vi "HEALTH_LABVIEW_V1.vi"() -> (0 "error out":errorcluster)   [LabVIEW 2026]
panel:
  in  "HEATER ON/OFF":bool
  out "ANALOG VOLTAGE 5\nADDRESS 8:\nHEATER TEMPERATURE":dbl(knob) scale=0.0..2.5
  out "Value 5":dbl format="%.6f"
  out "HEATER TEMP (C)":dbl(graph)
  out "ANALOG VOLTAGE 4\nADDRESS 22:\nCOOLANT OUTLET TEMPERATURE":dbl(knob) scale=0.0..2.5
  out "Value 4":dbl format="%.6f"
  out "ANALOG VOLTAGE 3\nADDRESS 20:\nCOOLANT INLET TEMPERATURE":dbl(knob) scale=0.0..2.5
  out "Value 3":dbl format="%.6f"
  out "ANALOG VOLTAGE 2\nADDRESS 18:\nDIFFERENTIAL PRESSURE":dbl(knob) scale=0.0..2.5
  out "Value 2":dbl format="%.6f"
  out "ANALOG VOLTAGE 1\nADDRESS 16:\nABSOLUTE PRESSURE":dbl(knob) scale=0.0..2.5
  out "Error String":string
  out "Value":dbl format="%.6f"
  out "ConnectionType Out":i32
  out "DeviceType Out":i32
  in  "Identifier":string="LJM_idANY"
  in  "ConnectionType":string="LJM_ctANY"
  in  "DeviceType":string="LJM_dtANY"
  # "LJM_dtT4"
  # "LJM_ctUSB"
  # "Common Registers:\nAddress, Name, Type, Read/Write\n0, AIN0, 3, RO\n2, AIN1, 3, RO\n1000, DAC0, 3, RW\n1002, DAC1, 3, RW\n2000, FIO0, 0, RW\n2001, FIO1, 0, RW\n55110, TEST_UINT16, 0, RW\n60000, PRODUCT_ID, 3, RO\n60004, FIRMWARE_VERSION, 3, RO\n60028, SERIAL_NUMBER, 1, RO\n\nTypes: 0=UINT16, 1=UINT32, 2=INT32, 3=FLOAT32"
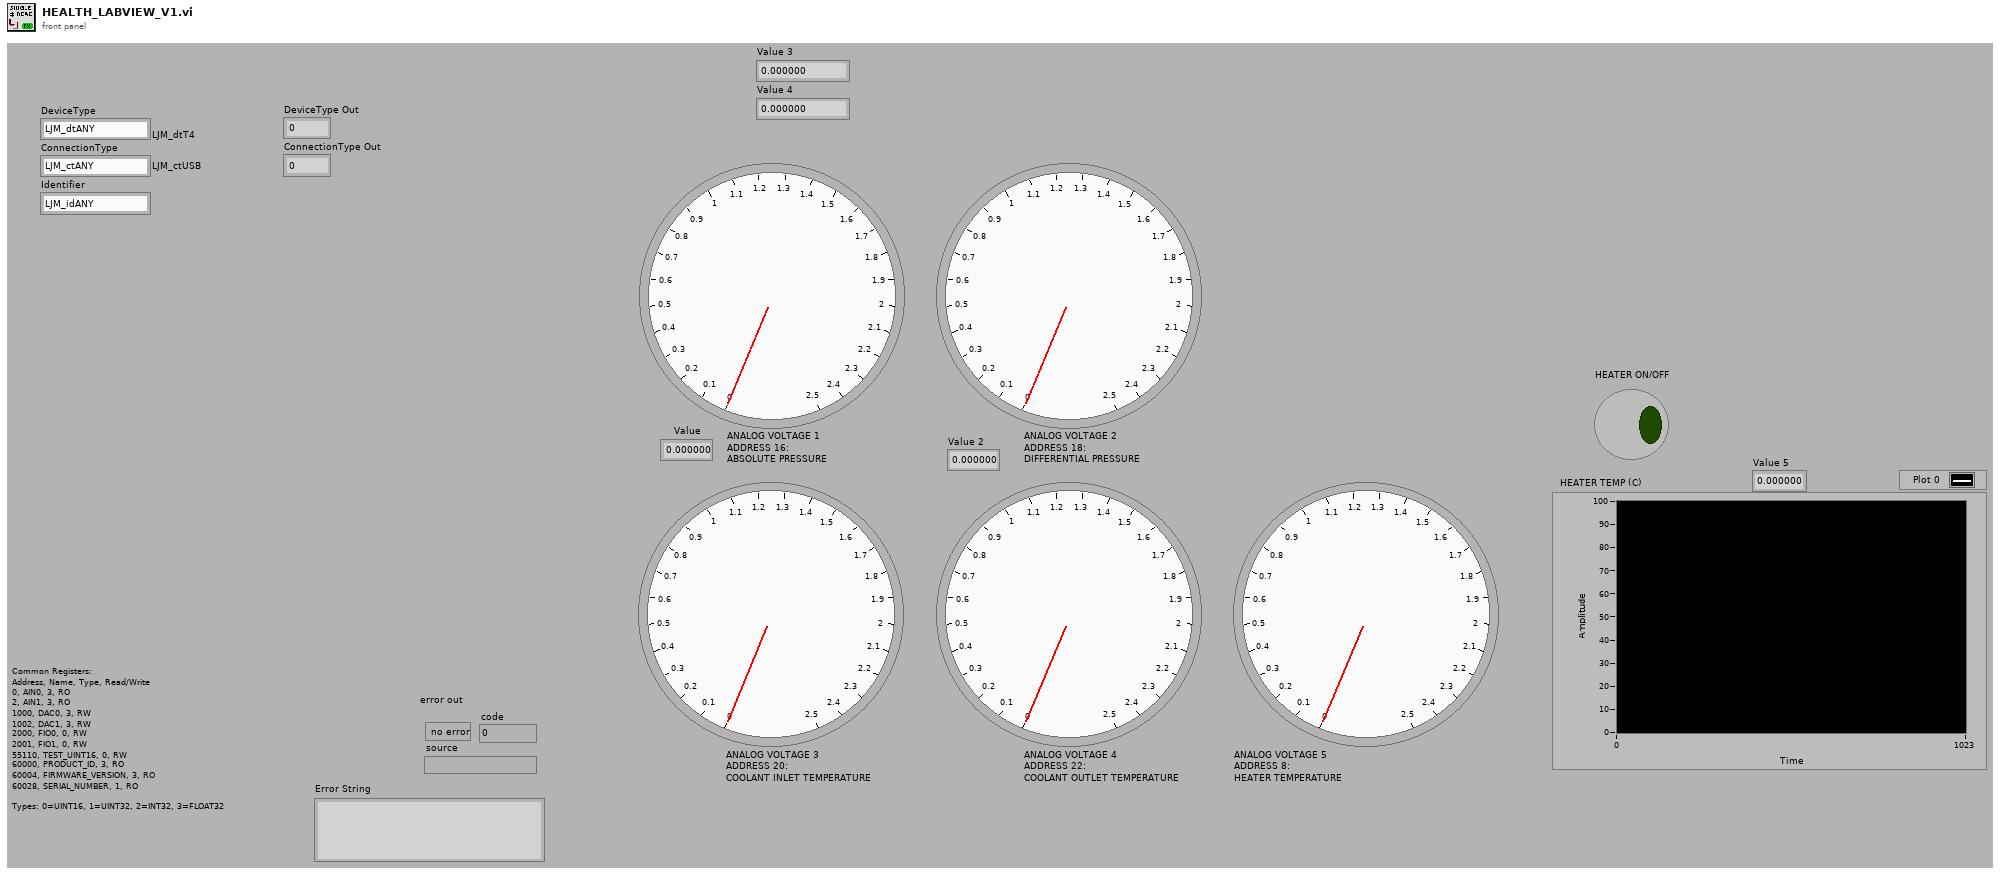
[diagram p1: front panel]
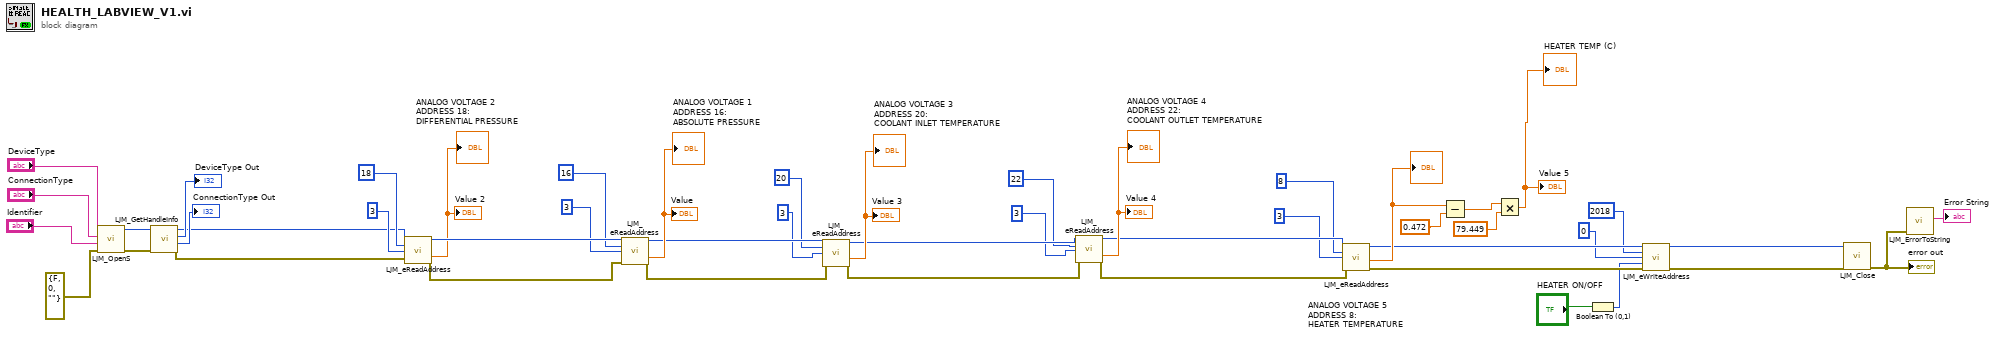
[diagram p0: block diagram]
diagram:
  n1 = call "LJM_OpenS.vi"("error in"=errorcluster {"status"=FALSE, "code"=0, "source"=""} ("error in (no error)"), "Identifier"="Identifier", "ConnectionType"="ConnectionType", "DeviceType"="DeviceType") -> ("error out"=w46:errorcluster, "Handle"=w45:i32)  [unwired: 6 in]
  n2 = call "LJM_GetHandleInfo.vi"("error in"=w46, "Handle In"=w45) -> ("error out"=w33:errorcluster, "ConnectionType"=→"ConnectionType Out":i32, "DeviceType"=→"DeviceType Out":i32, "Handle Out"=w34:i32)  [unwired: 2 in, 4 out]
  n3 = call "LJM_eReadAddress.vi"("Handle In"=w34, "Address"=18 ("Address 2"), "Type"=3 ("Type 2"), "error in"=w33) -> ("Handle Out"=w32:i32, "Value"=→"Value 2" →"ANALOG VOLTAGE 2\nADDRESS 18:\nDIFFERENTIAL PRESSURE":dbl, "error out"=w31:errorcluster)  [unwired: 9 in]
  n4 = call "LJM_eReadAddress.vi"("Handle In"=w32, "Address"=16 ("Address 2"), "Type"=3 ("Address 2"), "error in"=w31) -> ("Handle Out"=w28:i32, "Value"=→"Value" →"ANALOG VOLTAGE 1\nADDRESS 16:\nABSOLUTE PRESSURE":dbl, "error out"=w27:errorcluster)  [unwired: 9 in]
  n5 = call "LJM_eReadAddress.vi"("Handle In"=w28, "Address"=20 ("Address 2"), "Type"=3 ("Address 2"), "error in"=w27) -> ("Handle Out"=w26:i32, "Value"=→"Value 3" →"ANALOG VOLTAGE 3\nADDRESS 20:\nCOOLANT INLET TEMPERATURE":dbl, "error out"=w25:errorcluster)  [unwired: 9 in]
  n6 = call "LJM_eReadAddress.vi"("Handle In"=w26, "Address"=22 ("Address 2"), "Type"=3 ("Address 2"), "error in"=w25) -> ("Handle Out"=w23:i32, "Value"=→"Value 4" →"ANALOG VOLTAGE 4\nADDRESS 22:\nCOOLANT OUTLET TEMPERATURE":dbl, "error out"=w22:errorcluster)  [unwired: 9 in]
  n7 = call "LJM_eReadAddress.vi"("Handle In"=w23, "Address"=8 ("Address 2"), "Type"=3 ("Address 2"), "error in"=w22) -> ("Handle Out"=w8:i32, "Value"=w9:dbl, "error out"=w7:errorcluster)  [unwired: 9 in]
  "ANALOG VOLTAGE 5\nADDRESS 8:\nHEATER TEMPERATURE" <- w9
  n8 = Subtract(x=w9, y=0.472 ("Address 2")) -> (x-y=w12:dbl)
  n9 = Multiply(x=w12, y=79.449 ("Address 2")) -> (x*y=→"HEATER TEMP (C)" →"Value 5":dbl)
  n10 = Boolean To (0,1)(Boolean="HEATER ON/OFF") -> (0, 1=w1:i16)
  n11 = call "LJM_eWriteAddress.vi"("Handle In"=w8, "Address"=2018 ("Address 2"), "Type"=0 ("Address 2"), "Value"=w1, "error in"=w7) -> ("Handle Out"=w5:i32, "error out"=w6:errorcluster)  [unwired: 9 in]
  n12 = call "LJM_Close.vi"("error in"=w6, "Handle"=w5) -> ("error out"=w37:errorcluster)  [unwired: 9 in]
  "error out" <- w37
  n13 = call "LJM_ErrorToString.vi"("error in"=w37) -> ("String"=→"Error String":string)  [unwired: 10 in]
